vi "Do Something Else and Wait for Reply.vi"(8 "error in (no error)":errorcluster, 9 "X":dbl, 10 "Do Something Else Message":string, 11 "Module ID":i32=-1) -> (0 "error out":errorcluster, 1 "timed out?":bool, 2 "Reply Payload":T1)   [LabVIEW 2017, in "My Cloneable Module.lvlib"]
doc: "Send the Do Something Else request to the Module's Main.vi.\n_____\nBased on Delacor QMH Project Template 3.1.0.34."
uses:
  My Cloneable Module.lvlib
  Do Something Else and Wait (Reply Payload)--cluster.ctl
  Do Something Else and Wait for Reply Argument--cluster.ctl
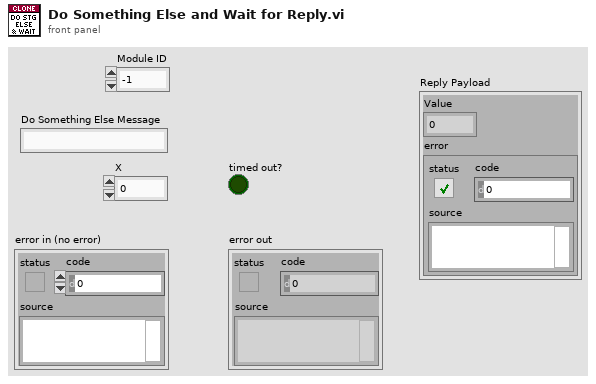
[diagram p1: front panel]
types:
  T1 = typedef "My Cloneable Module.lvlib/Do Something Else and Wait (Reply Payload)--cluster.ctl" = cluster{"Value":dbl, "error":errorcluster}
  T2 = typedef "My Cloneable Module.lvlib/Request Events--cluster.ctl" = cluster{"Stop Module":refnum<user-event>, "Do Something":refnum<user-event>, "Do Something Else":refnum<user-event>, "Do Something Else and Wait for Reply":refnum<user-event>, "Show Panel":refnum<user-event>, "Hide Panel":refnum<user-event>, "Show Diagram":refnum<user-event>, "Get Module Execution Status":refnum<user-event>}
  T3 = typedef "My Cloneable Module.lvlib/Do Something Else and Wait for Reply Argument--cluster.ctl" = cluster{"Do Something Else Msg":string, "X":dbl, "Wait Notifier":refnum<notifier>, "Module ID":i32}
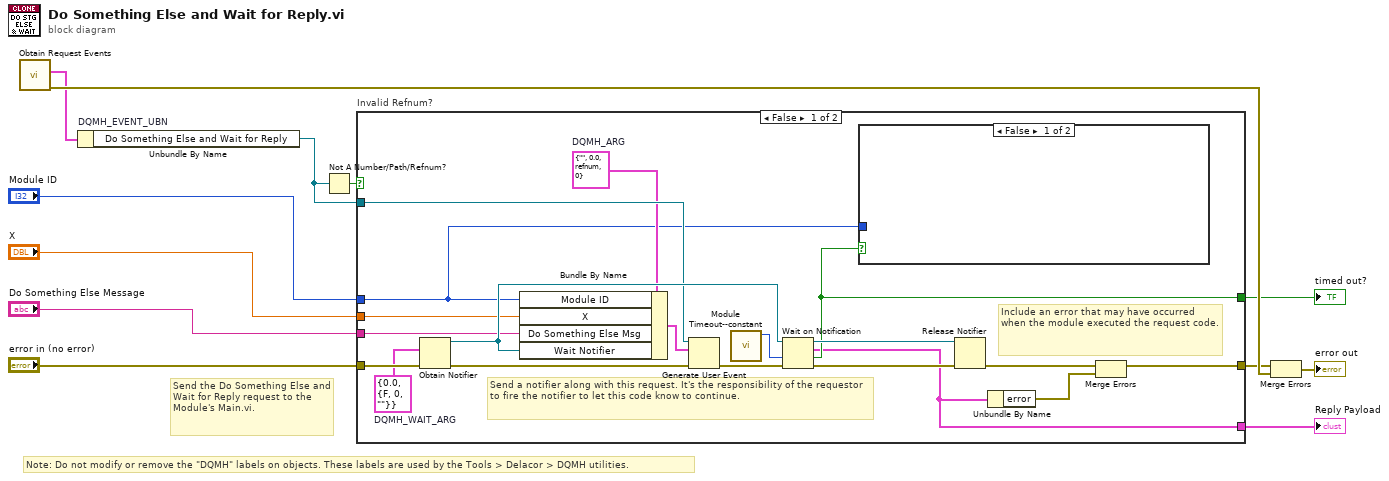
[diagram p0: block diagram]
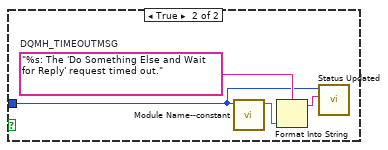
[diagram p2: hidden frame]
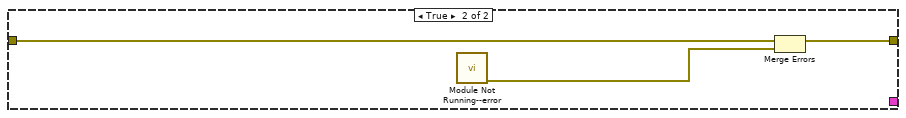
[diagram p3: hidden frame]
diagram:
  # "Note: Do not modify or remove the \"DQMH\" labels on objects. These labels are used by the Tools > Delacor > DQMH utilities."
  # "Send the Do Something Else and Wait for Reply request to the Module's Main.vi."
  n1 = call "Obtain Request Events.vi"() -> ("error out"=w11:errorcluster, "My Cloneable Module Request Events"=w10:T2)  [unwired: 10 in]
  n2 = Unbundle By Name "DQMH_EVENT_UBN"(w10) -> ("Do Something Else and Wait for Reply"=w8:refnum<user-event>)
  n3 = Not A Number/Path/Refnum?(number/path/refnum=w8) -> (NaN/Path/Refnum?=w9:bool)
  n4 = case "Invalid Refnum?" shown="False" w9 {
    tunnel: [w15 w37] -> w4
    tunnel: "X" -> [w24 _]
    tunnel: "Do Something Else Message" -> [w23 _]
    tunnel: "error in (no error)" -> [w22 w36]
    tunnel: w8 -> [w20 _]
    tunnel: "Module ID" -> [w18 _]
    tunnel: [w16 _] -> w2
    tunnel: [w14 _] -> w1
    frame False {
      w17 = T1 {"Value"=0.0, "error"={"status"=FALSE, "code"=0, "source"=""}}  # DQMH_WAIT_ARG
      w19 = T3 {"Do Something Else Msg"="", "X"=0.0, "Wait Notifier"=refnum, "Module ID"=0}  # DQMH_ARG
      # "Include an error that may have occurred when the module executed the request code."
      # "Send a notifier along with this request. It's the responsibility of the requestor to fire the notifier to let this code know to continue."
      n5 = Obtain Notifier(notification data type=w17, error in (no error)=w22) -> (notifier out=w27:refnum<notifier>, error out=w28:errorcluster)  [unwired: 2 in, 1 out]
      n6 = Bundle By Name(cluster=w19, "Module ID"=w18, "X"=w24, "Do Something Else Msg"=w23, "Wait Notifier"=w27) -> (w29:T3)
      n7 = Generate User Event(user event=w20, event data cluster=w29, error in=w28) -> (error out=w30:errorcluster)  [unwired: 1 in, 1 out]
      n8 = call "Module Timeout--constant.vi"() -> ("Module Timeout"=w26:i32)  [unwired: 11 in]
      n9 = Wait on Notification(notifier=w27, timeout in ms (-1)=w26, error in (no error)=w30) -> (notifier out=w25:refnum<notifier>, notification=w14:T1, timed out?=w16:bool, error out=w31:errorcluster)  [unwired: 1 in]
      n10 = case shown="False" w16 {
        tunnel: w18 -> [_ w32]
        frame False {
        }
        frame True {
          w33 = "%s: The 'Do Something Else and Wait for Reply' request timed out."  # DQMH_TIMEOUTMSG
          n11 = call "Module Name--constant.vi"("Module ID"=w32) -> ("Module Name"=w34:string)  [unwired: 10 in]
          n12 = Format Into String(format string=w33, w34) -> (resulting string=w35:string)  [unwired: 2 in, 1 out]
          n13 = call "Status Updated.vi"("Status"=w35, "Module ID"=w32) -> ()  [unwired: 9 in, 1 out]
        }
      }
      n14 = Release Notifier(notifier=w25, error in (no error)=w31) -> (error out=w21:errorcluster)  [unwired: 1 in, 2 out]
      n15 = Unbundle By Name(w14) -> ("error"=w13:errorcluster)
      n16 = Merge Errors(w21, w13) -> (w15:errorcluster)
    }
    frame True {
      n17 = call "Module Not Running--error.vi"() -> ("error out"=w38:errorcluster)  [unwired: 11 in]
      n18 = Merge Errors(w36, w38) -> (w37:errorcluster)
    }
  }
  "timed out?" <- w2
  "Reply Payload" <- w1
  n19 = Merge Errors(w4, w11) -> (→"error out":errorcluster)
